vi "E441X_PM_Configure_Trigger.vi"(0 "VISA session":refnum<visa-resource-name>, 1 "Channel (0: A)":i32(ring) items=["A", "B"], 5 "Delay Auto State (T: On)":bool=TRUE, 7 "Source (0: Immediate)":i32(ring) items=["Immediate", "Bus", "Hold", "External", "Internal A", "Internal B"], 11 "error in (no error)":errorcluster {"code" format="%.0x"}) -> (4 "dup VISA session":refnum<visa-resource-name>, 15 "error out":errorcluster {"code" format="%.0x"})   [LabVIEW 2015]
doc: "This VI configures the trigger system."
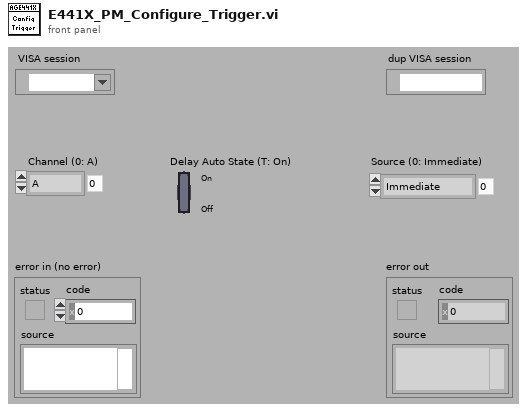
[diagram p1: front panel]
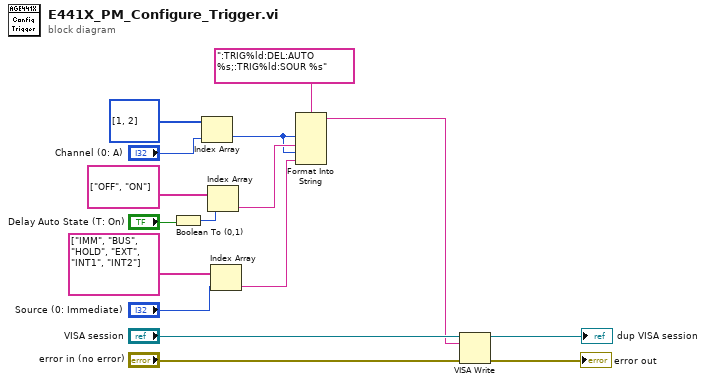
[diagram p0: block diagram]
diagram:
  n1 = Boolean To (0,1)(Boolean="Delay Auto State (T: On)") -> (0, 1=w10:i16)
  n2 = Index Array(array=i32[] [1, 2], index="Channel (0: A)") -> (element=w7:i32)
  n3 = Index Array(array=string[] ["OFF", "ON"], index=w10) -> (element=w8:string)
  n4 = Index Array(array=string[] ["IMM", "BUS", "HOLD", "EXT", "INT1", "INT2"], index="Source (0: Immediate)") -> (element=w4:string)
  n5 = Format Into String(format string=":TRIG%ld:DEL:AUTO %s;:TRIG%ld:SOUR %s", w7, w8, w7, w4) -> (resulting string=w3:string)  [unwired: 2 in, 1 out]
  n6 = VISA Write(VISA resource name="VISA session", write buffer=w3, error in (no error)="error in (no error)") -> (VISA resource name out=→"dup VISA session":refnum<visa-resource-name>, error out=→"error out":errorcluster)  [unwired: 1 out]
